vi "测试matlab文件读取轨迹矩阵.vi"() -> ()   [LabVIEW 2018]
panel:
  in  "停止":bool
  out "Real 2":dbl
  out "Real":dbl
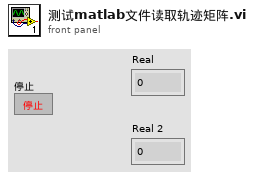
[diagram p1: front panel]
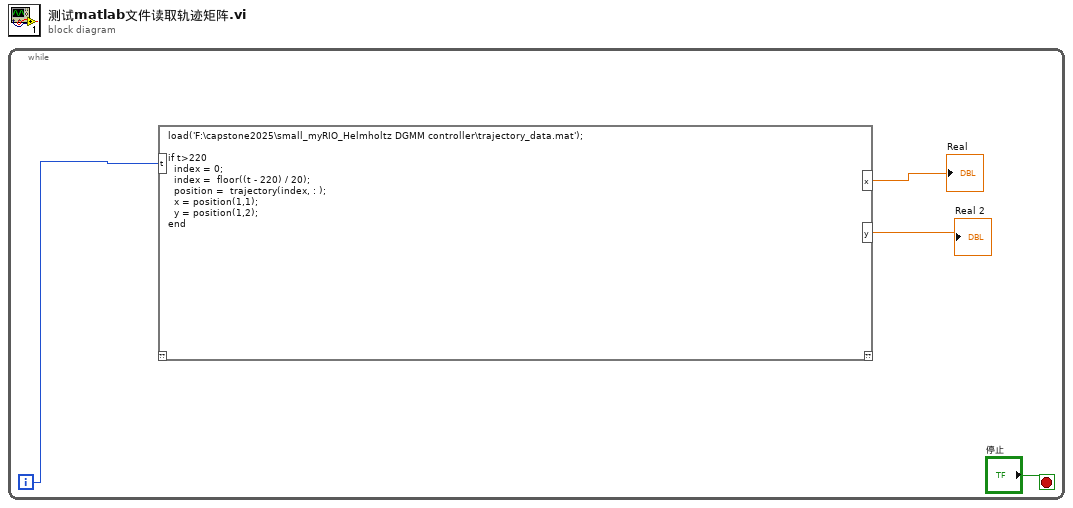
[diagram p0: block diagram]
diagram:
  n1 = while {
    i -> [w2]
    stop <- "停止" stop-if-true
    n2 = script code="load('F:\\capstone2025\\small_myRIO_Helmholtz DGMM controller\\trajectory_data.mat');\n\nif t>220 \n  index = 0;\n  index =  floor((t - 220) / 20);\n  position =  trajectory(index, : );\n  x = position(1,1);\n  y = position(1,2);\nend"("t"=w2) -> ("x"=→"Real":dbl, "y"=→"Real 2":dbl)  [unwired: 1 in, 1 out]
  }
